vi "Test Coffee Shop Added Customer Broadcasts Status.vi"(8 "error in (no error)":errorcluster, 11 "Coffee Shop Test In":refnum<class "Coffee Shop Test.lvclass">) -> (0 "error out":errorcluster, 3 "Coffee Shop Test Out":refnum<class "Coffee Shop Test.lvclass">)   [LabVIEW 2020, in "Coffee Shop Test.lvclass"]
uses:
  Coffee Shop Test.lvclass
  C:/Program Files (x86)/National Instruments/LabVIEW 2020/vi.lib/Asteme/LUnit/Test Case.lvclass
  Processes/Coffee Shop/Coffee Shop.lvclass
  C:/Program Files (x86)/National Instruments/LabVIEW 2020/vi.lib/Asteme/Triarc Framework/Process/Process.lvclass
  C:/Program Files (x86)/National Instruments/LabVIEW 2020/vi.lib/Asteme/Triarc Framework/Application/Application.lvclass
  <vilib>/Asteme/Triarc Framework/Process/Process.lvclass/Process.ctl
  <vilib>/Asteme/LUnit/Test Case.lvclass/Test Case.ctl
  <vilib>/Asteme/LUnit/LUnit Assertion Result.lvclass/LUnit Assertion Result.ctl
  <vilib>/Asteme/Triarc Framework/Broadcast Event Helpers/Execution timer.vi
  <vilib>/Asteme/Triarc Framework/Process/Protected/Messaging/Enqueue Message.vi
  <vilib>/Asteme/Triarc Framework/Process/Private/SubVIs/Wait for finish.vi
  <vilib>/Asteme/Triarc Framework/Process/Private/SubVIs/Set Lifecycle State.vi
  <vilib>/Asteme/Triarc Framework/Process/Public/Lifecycle/Get Lifecycle State.vi
  <vilib>/Asteme/LUnit/Palette/Pass If.vi
  <vilib>/Asteme/LUnit/Set Assertion Type.vi
  <vilib>/Utility/error.llb/Clear Errors.vi
  <vilib>/Asteme/LUnit/Palette/Fail.vi
  <vilib>/Asteme/LUnit/Palette/Pass.vi
  <vilib>/Asteme/LUnit/LUnit Write Assertion Type.vi
  <vilib>/Asteme/LUnit/Add test result.vi
  <vilib>/Asteme/LUnit/LUnit Write Passed.vi
  <vilib>/Asteme/LUnit/LUnit Get Test Case.vi
  <vilib>/Asteme/LUnit/Assertion Result/LUnit Get Test Name.vi
  <vilib>/Asteme/LUnit/LUnit Write Message.vi
  <vilib>/Asteme/LUnit/LUnit Write Description.vi
  <vilib>/Asteme/LUnit/Read Test Case Name.vi
  <vilib>/Asteme/Triarc Framework/Broadcast Event Helpers/Dequeue Broadcast Message.vi
  <vilib>/Utility/error.llb/Error Cluster From Error Code.vi
  <vilib>/Asteme/LUnit/LUnit Assertion Result.lvclass
  <vilib>/Asteme/Triarc Framework/Application/Application.lvclass
  <vilib>/Asteme/Triarc Framework/Process/Process.lvclass
  <vilib>/Asteme/LUnit/Test Case.lvclass
  <vilib>/Asteme/Triarc Framework/Broadcast Event Helpers/Broadcast Event Helpers.lvlib
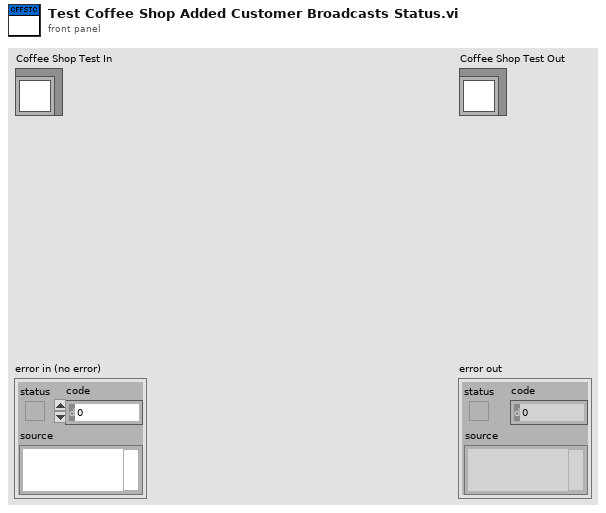
[diagram p1: front panel]
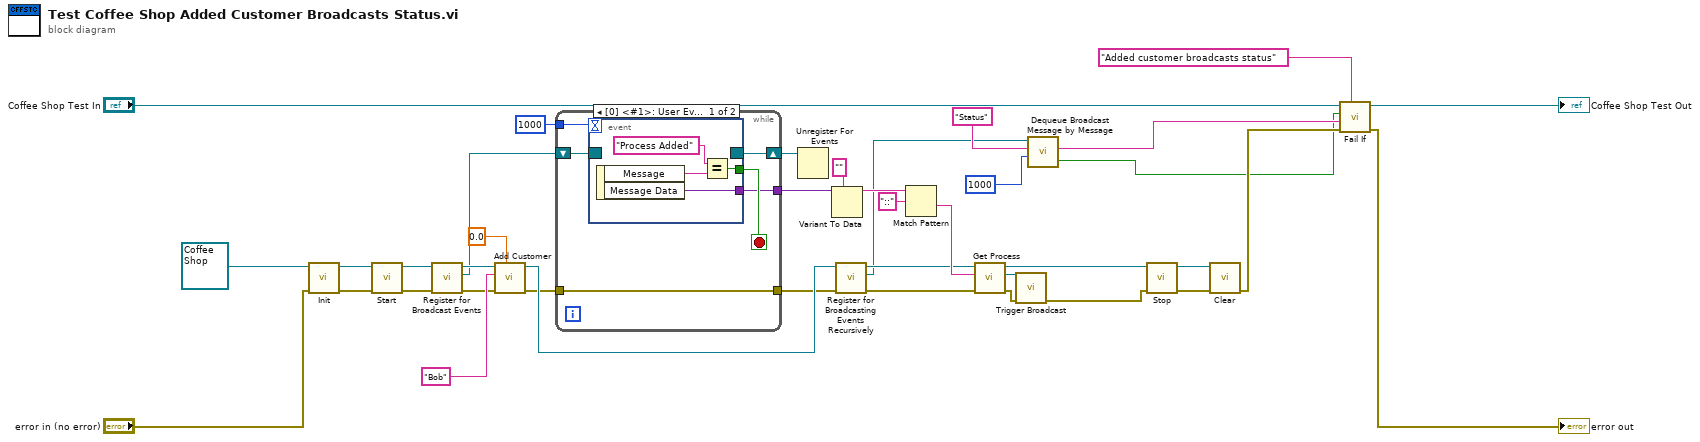
[diagram p0: block diagram]
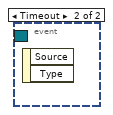
[diagram p2: hidden frame]
diagram:
  n1 = call-dynamic "Init.vi"("error in (no error)"="error in (no error)", "Process In"=refnum<class "Coffee Shop.lvclass"> refnum ("Coffee Shop.lvclass")) -> ("error out"=w37:errorcluster, "Process Out"=w38:refnum<class "Coffee Shop.lvclass">)  [unwired: 8 in]
  n2 = call <vilib>:"Start.vi"("error in (no error)"=w37, "Process In"=w38) -> ("error out"=w22:errorcluster, "Process Out"=w23:refnum<class "Coffee Shop.lvclass">)  [unwired: 8 in]
  n3 = call <vilib>:"Register for Broadcast Events.vi"("error in (no error)"=w22, "Process In"=w23) -> ("error out"=w20:errorcluster, "Event Registration Refnum Out"=w19:refnum<event-registration>, "Process Out"=w21:refnum<class "Coffee Shop.lvclass">)  [unwired: 7 in]
  n4 = call "Add Customer.vi"("Time scale [ms]"=0.0 ("Delay Before Leaving [s]"), "error in (no error)"=w20, "Name"="Bob", "Coffee Shop in"=w21) -> ("error out"=w3:errorcluster, "Coffee Shop out"=w7:refnum<class "Coffee Shop.lvclass">)  [unwired: 6 in]
  n5 = while {
    shift-right: [w44] -> w18
    shift-left: w19 -> [w45]
    tunnel: 1000 -> [w43]
    tunnel: [w41] -> w16
    tunnel: [w40] -> w4
    tunnel: w3 -> [w40]
    stop <- w42 stop-if-true
    n6 = event shown="[0] <#1>: User Event" {
      selector: w45 -> [_ _]
      dyn-events: [_ _] -> w44
      timeout: w43 -> [_ _]
      tunnel: [w47 _] -> w42
      tunnel: [w46 _] -> w41
      event User Event {
        n7 = event-data() -> ("Message"=w49:string, "Message Data"=w46:variant)  [unwired: 1 in]
        n8 = Equal?(x="Process Added", y=w49) -> (x = y?=w47:bool)
      }
      event Timeout {
        n9 = event-data() -> ()  [unwired: 1 in, 2 out]
      }
    }
  }
  n10 = Unregister For Events(event registration refnum=w18) -> ()  [unwired: 1 in, 1 out]
  n11 = Variant To Data(type="", Variant=w16) -> (data=w13:string)  [unwired: 1 in, 1 out]
  n12 = call <vilib>:"Register for Broadcasting Events Recursively.vi"("error in (no error)"=w4, "Application In"=w7) -> ("error out"=w5:errorcluster, "Event Registration Refnum Out"=w2:refnum<event-registration>, "Application Out"=w6:refnum<class "Coffee Shop.lvclass">)  [unwired: 7 in]
  n13 = Match Pattern(string=w13, regular expression="::") -> (after substring=w10:string)  [unwired: 1 in, 3 out]
  n14 = call <vilib>:"Get Process.vi"("error in (no error)"=w5, "Process Name"=w10, "Rig In"=w6) -> ("error out"=w15:errorcluster, "App Process"=w8:refnum<class "Process.lvclass">, "Rig Out"=w14:refnum<class "Coffee Shop.lvclass">)  [unwired: 6 in]
  n15 = call <vilib>:"Trigger Broadcast.vi"("error in (no error)"=w15, "Process in"=w8) -> ("error out"=w9:errorcluster)  [unwired: 8 in, 1 out]
  n16 = call <vilib>:"Dequeue Broadcast Message by Message.vi"("Timeout (-1)"=1000, "Message"="Status", "Event Registration Refnum"=w2) -> ("Message"=w25:string, "Timed Out?"=w24:bool)  [unwired: 4 in, 3 out]
  n17 = call <vilib>:"Stop.vi"("error in (no error)"=w9, "Process In"=w14) -> ("error out"=w35:errorcluster, "Process Out"=w36:refnum<class "Coffee Shop.lvclass">)  [unwired: 7 in, 1 out]
  n18 = call-dynamic "Clear.vi"("error in (no error)"=w35, "Application In"=w36) -> ("error out"=w31:errorcluster)  [unwired: 9 in]
  n19 = call <vilib>:"Fail If.vi"("Description"="Added customer broadcasts status", "error in (no error)"=w31, "Message"=w25, "Fail?"=w24, "Test Case In"="Coffee Shop Test In") -> ("error out"=→"error out":errorcluster, "Test Case Out"=→"Coffee Shop Test Out":refnum<class "Coffee Shop Test.lvclass">)  [unwired: 5 in]
